vi "NF WF1973_74 PSC.vi"(6 "Read(F)":bool, 8 "error in (no error)":errorcluster caption="Error IN", 10 "Clear?(NO)":bool, 11 "VISAsession":refnum<visa-resource-name>) -> (0 "error out":errorcluster caption="Error OUT", 2 "Query PSC":i32=9, 3 "CopyVISAsession":refnum<visa-resource-name>)   [LabVIEW 2010]
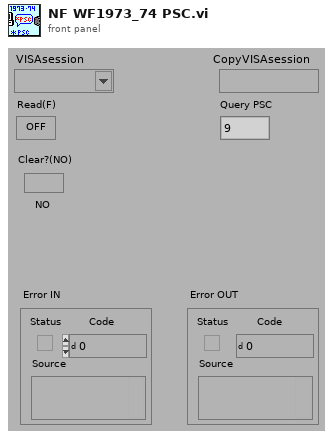
[diagram p1: front panel]
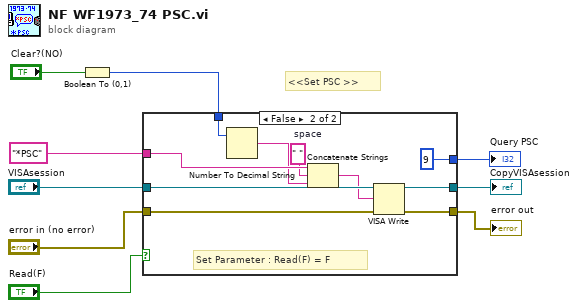
[diagram p0: block diagram]
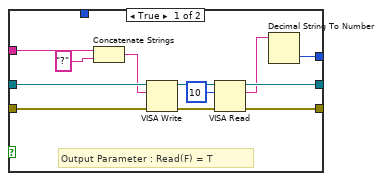
[diagram p2: hidden frame]
diagram:
  # "<<Set PSC >>"
  n1 = Boolean To (0,1)(Boolean="Clear?(NO)") -> (0, 1=w1:i16)
  n2 = case shown="FALSE" "Read(F)" {
    tunnel: "VISAsession" -> [w21 w31]
    tunnel: [w12 w28] -> w8
    tunnel: [w18 w29] -> w7
    tunnel: "error in (no error)" -> [w17 w30]
    tunnel: "*PSC" ("文字列") -> [w15 w24]
    tunnel: [w10 9] -> w3
    tunnel: w1 -> [_ w26]
    frame True {
      # "Output Parameter : Read(F) = T"
      n3 = Concatenate Strings(w15, "?" ("形式文字列")) -> (w13:string)
      n4 = VISA Write(VISA resource name=w21, write buffer=w13, error in (no error)=w17) -> (VISA resource name out=w19:refnum<visa-resource-name>, error out=w20:errorcluster)  [unwired: 1 out]
      n5 = VISA Read(VISA resource name=w19, byte count=u32 10 ("バイトカウント（0）"), error in (no error)=w20) -> (VISA resource name out=w12:refnum<visa-resource-name>, read buffer=w11:string, error out=w18:errorcluster)  [unwired: 1 out]
      n6 = Decimal String To Number(string=w11) -> (number=w10:i32)  [unwired: 2 in, 1 out]
    }
    frame False {
      w22 = " "  # space
      # "Set Parameter : Read(F) = F"
      n7 = Number To Decimal String(number=w26) -> (decimal integer string=w23:string)  [unwired: 1 in]
      n8 = Concatenate Strings(w24, w22, w23) -> (w25:string)
      n9 = VISA Write(VISA resource name=w31, write buffer=w25, error in (no error)=w30) -> (VISA resource name out=w28:refnum<visa-resource-name>, error out=w29:errorcluster)  [unwired: 1 out]
    }
  }
  "error out" <- w7
  "CopyVISAsession" <- w8
  "Query PSC" <- w3
